vi "prob.vi"(11 "field":T1[][](array[typedef])) -> (3 "result":enum32{"black", "white", "none"}[][](array[radio]))   [LabVIEW 2022 SP3]
uses:
  moku.ctl
panel:
  out "Array":i32[][](array[numeric])
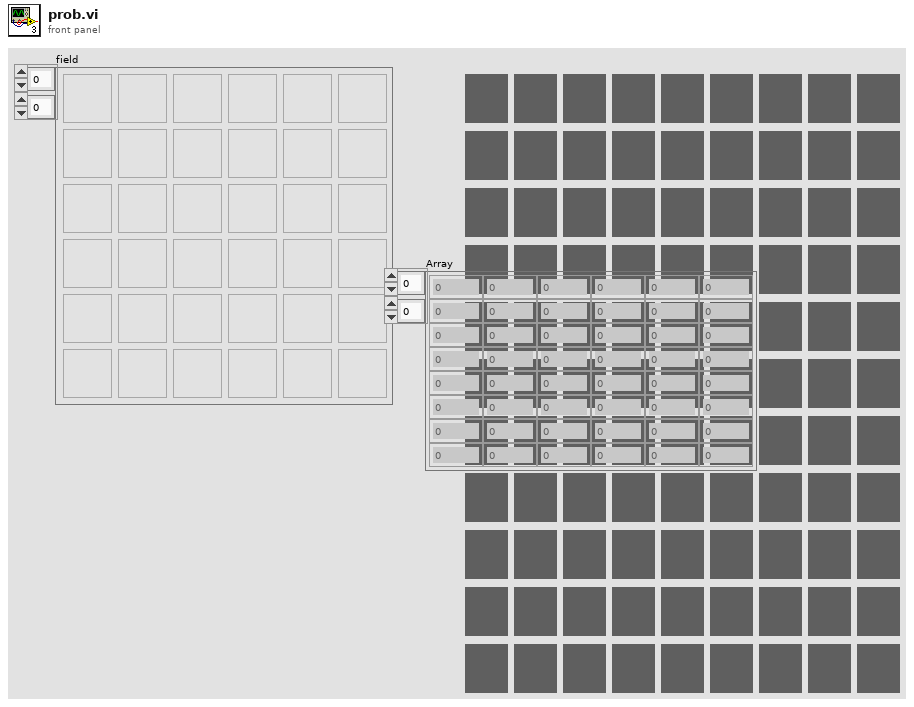
[diagram p1: front panel]
types:
  T1 = typedef "moku.ctl" = enum32{"90b", "70b", "30b", "10b", "none"}
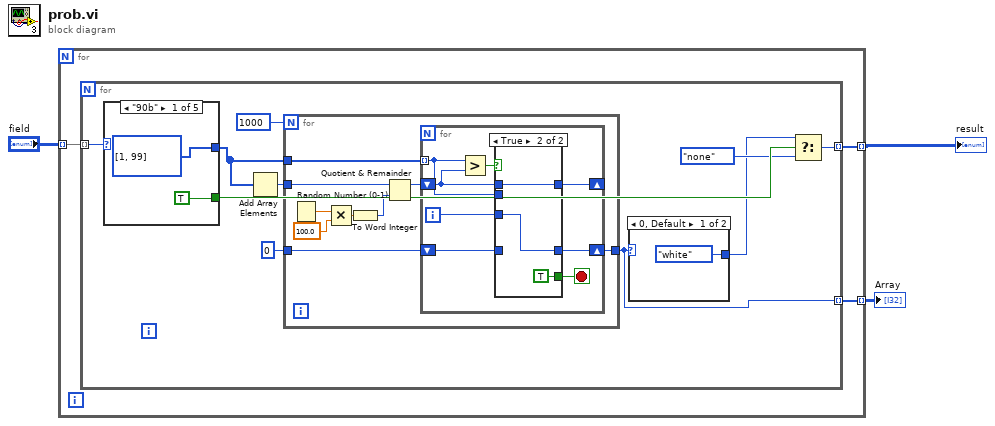
[diagram p0: block diagram]
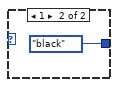
[diagram p2: hidden frame]
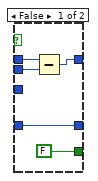
[diagram p3: hidden frame]
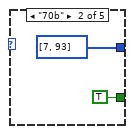
[diagram p4: hidden frame]
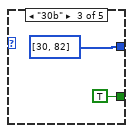
[diagram p5: hidden frame]
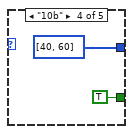
[diagram p6: hidden frame]
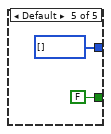
[diagram p7: hidden frame]
diagram:
  n1 = for {
    tunnel: "field" -> [w6] mode=indexing
    tunnel: [w5] -> w2 mode=indexing
    tunnel: [w4] -> w1 mode=indexing
    n2 = for {
      tunnel: w6 -> [w16] mode=indexing
      tunnel: [w9] -> w5 mode=indexing
      tunnel: [w8] -> w4 mode=indexing
      n3 = case shown="\"90b\"" w16 {
        tunnel: [i16[] [1, 99] ("90") i16[] [7, 93] ("70") i16[] [30, 82] ("30") i16[] [40, 60] ("10") i16[] [] ("10")] -> w13
        tunnel: [TRUE TRUE TRUE TRUE FALSE] -> w11
        frame "90b" {
        }
        frame "70b" {
        }
        frame "30b" {
        }
        frame "10b" {
        }
        frame Default {
        }
      }
      n4 = Add Array Elements(numeric array=w13) -> (sum=w15:i16)
      n5 = for {
        N: 1000 -> [_]
        tunnel: w13 -> [w27]
        tunnel: 0 ("pick") -> [w25]
        tunnel: [w26] -> w8
        tunnel: w15 -> [w20]
        n6 = Random Number (0-1)() -> (number: 0 to 1=w23:dbl)
        n7 = Multiply(x=w23, y=100.0 ("x")) -> (x*y=w24:dbl)
        n8 = To Word Integer(number=w24) -> (16bit integer=w21:i16)
        n9 = Quotient & Remainder(x=w20, y=w21) -> (x-y*floor(x/y)=w19:i16)  [unwired: 1 out]
        n10 = for {
          tunnel: w27 -> [w28] mode=indexing
          shift-right: [w34] -> w26
          shift-left: w25 -> [w32]
          shift-right: [w30] -> _
          shift-left: w19 -> [w29]
          i -> [w33]
          stop <- w31 stop-if-true
          n11 = Greater?(x=w28, y=w29) -> (0:w35:bool)
          n12 = case shown="True" w35 {
            tunnel: [w40 w43] -> w34
            tunnel: w33 -> [_ w43]
            tunnel: w32 -> [w40 _]
            tunnel: [FALSE TRUE] -> w31
            tunnel: [w36 w41] -> w30
            tunnel: w29 -> [w38 w41]
            tunnel: w28 -> [w37 _]
            frame False {
              n13 = Subtract(x=w38, y=w37) -> (x-y=w36:i16)
            }
            frame True {
            }
          }
        }
      }
      n14 = case shown="0, Default" w8 {
        tunnel: [enum32{"black", "white", "none"}."white" ("black/white") enum32{"black", "white", "none"}."black" ("black/white")] -> w7
        frame 0, Default {
        }
        frame 1 {
        }
      }
      n15 = Select(t=w7, s=w11, f=enum32{"black", "white", "none"}."none" ("black/white")) -> (s? t:f=w9:enum32{"black", "white", "none"})
    }
  }
  "result" <- w2
  "Array" <- w1
